vi "Compute.vi"(8 "error in (no error)":errorcluster, 9 "Data Channels":T3, 10 "x-var":T2(array[cluster]), 11 "Average in":refnum<class "Average.lvclass">) -> (0 "error out":errorcluster, 1 "Add'l Data Channels":T3, 3 "Average out":refnum<class "Average.lvclass">)   [LabVIEW 2017, in "Average.lvclass"]
doc: "Given a data channel and an x-coordinate, compute and return one or more new data channels."
uses:
  Average.lvclass
  Instruments/Utility Classes/Readable/Data Channels.ctl
  Instruments/Utility Classes/Readable/Data Channel.ctl
  Instruments/Utility Classes/Readable/Data Point.ctl
  Instruments/Utility Classes/Readable/Time.ctl
  Instruments/Utility Classes/Readable/X.ctl
  Instruments/Utility Classes/Readable/Readable.lvclass
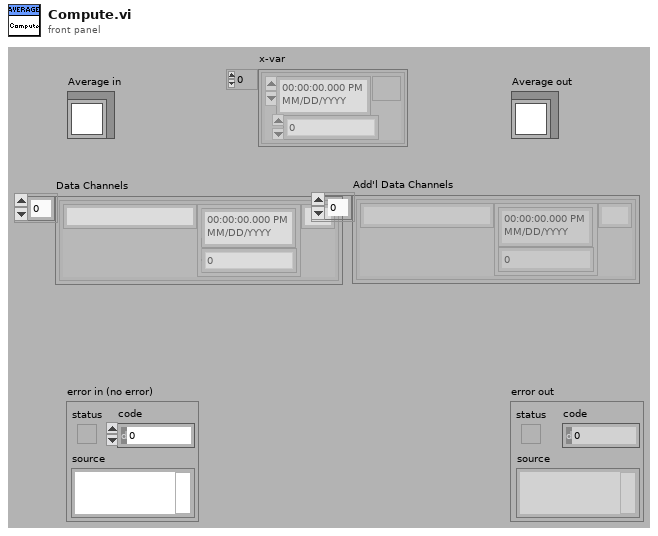
[diagram p1: front panel]
types:
  T1 = typedef "Readable.lvclass/X.ctl" = dbl
  T2 = cluster{"seconds since 1Jan1904":timestamp, "X-Var":T1}[]
  T3 = typedef "Readable.lvclass/Data Channels.ctl" = T4[]
  T4 = typedef "Readable.lvclass/Data Channel.ctl" = cluster{"Name":string, "Data Point":T5, "Unit":string}
  T5 = typedef "Readable.lvclass/Data Point.ctl" = cluster{"t":T6, "x":T1}
  T6 = typedef "Readable.lvclass/Time.ctl" = timestamp
  T7 = cluster{"seconds since 1Jan1904":timestamp, "x":T1}
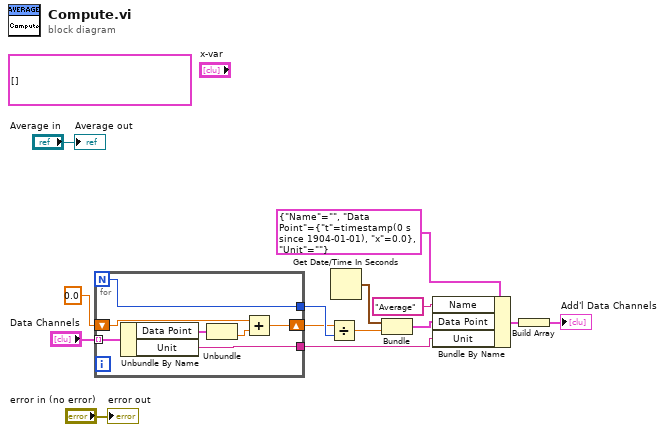
[diagram p0: block diagram]
diagram:
  (unwired) T3 [] ("Data Channels")
  n1 = for {
    N -> [w17]
    tunnel: "Data Channels" -> [w21] mode=indexing
    shift-right: [w19] -> w12
    shift-left: T1 0.0 ("x") -> [w18]
    tunnel: [w17] -> w13
    tunnel: [w16] -> w8
    n2 = Unbundle By Name(w21) -> ("Data Point"=w20:T5, "Unit"=w16:string)
    n3 = Unbundle(w20) -> ("x"=w15:T1)  [unwired: 1 out]
    n4 = Add(x=w18, y=w15) -> (x+y=w19:T1)
  }
  n5 = Divide(x=w12, y=w13) -> (x/y=w2:T1)
  n6 = Get Date/Time In Seconds() -> (seconds since 1Jan1904=w1:timestamp)
  n7 = Bundle("seconds since 1Jan1904"=w1, "x"=w2) -> (w3:T7)  [unwired: 1 in]
  n8 = Bundle By Name(cluster=T4 {"Name"="", "Data Point"={"t"=timestamp(0 s since 1904-01-01), "x"=0.0}, "Unit"=""} ("Data Channel"), "Name"="Average", "Data Point"=w3, "Unit"=w8) -> (w6:T4)
  n9 = Build Array(w6) -> (→"Add'l Data Channels":T4[])
  "error out" <- "error in (no error)"
  "Average out" <- "Average in"
